vi "Position_Two_ScoringB.vi"(11 "data string":string) -> (3 "String":string)   [LabVIEW 2012, in "Serenity_mk2.lvrbt"]
uses:
  Serenity_mk2.lvrbt
  auto_drive_TYP.ctl
  State_Typ.ctl
  <vilib>/NXT/Dual Mode Library/Sound/Tone.vi
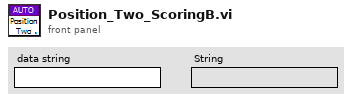
[diagram p1: front panel]
types:
  T1 = typedef "auto_drive_TYP.ctl" = cluster{"Left X":i8, "Left Y":i8, "Right Y":i8, "Power (100)":i8, "Wait (ms)":u32, "Enc/Deg Target":i32, "Move Type":enum16{"Relative Degrees", "Wait", "Encoder"}}
  T2 = typedef "State_Typ.ctl" = enum16{"Stop", "Check for Position 3", "Check for Position 2", "Move", "Reset Enc", "Read Enc", "Lift", "Dump Close"}
  T3 = typedef "LVHSConnector.ctl" = refnum<class "BrickReference.lvclass">
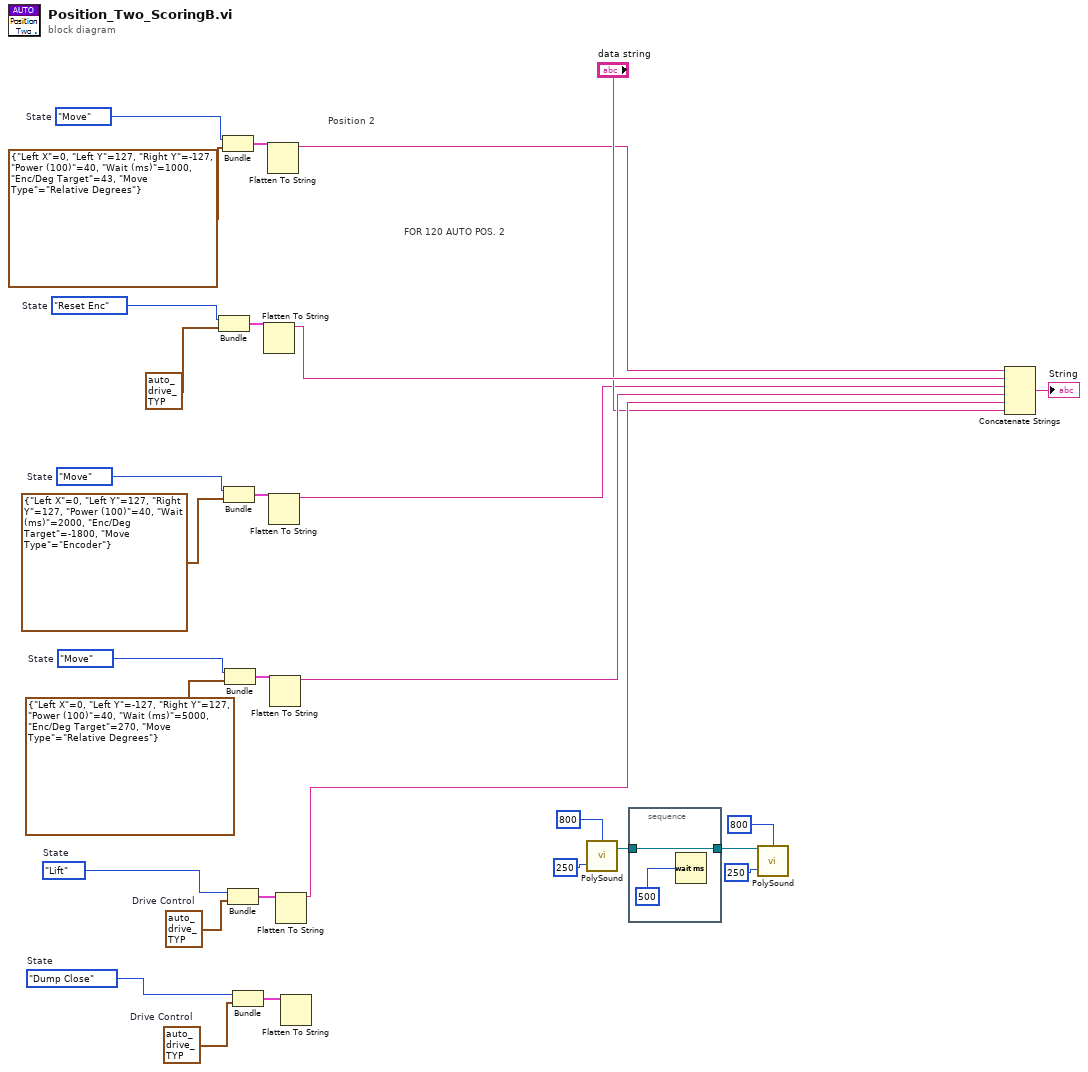
[diagram p0: block diagram]
diagram:
  w12 = T1 {"Left X"=0, "Left Y"=0, "Right Y"=0, "Power (100)"=100, "Wait (ms)"=3000, "Enc/Deg Target"=8450, "Move Type"=enum."Encoder"}  # Drive Control
  w13 = T1 {"Left X"=0, "Left Y"=0, "Right Y"=0, "Power (100)"=40, "Wait (ms)"=0, "Enc/Deg Target"=-6500, "Move Type"=enum."Encoder"}  # Drive Control
  w26 = State_Typ."Reset Enc"  # State
  w14 = State_Typ."Dump Close"  # State
  w10 = State_Typ."Lift"  # State
  w9 = State_Typ."Move"  # State
  w6 = State_Typ."Move"  # State
  w3 = State_Typ."Move"  # State
  # "FOR 120 AUTO POS. 2"
  # "Position 2"
  n1 = Bundle("State"=w26, "Drive Control"=T1 {"Left X"=0, "Left Y"=127, "Right Y"=127, "Power (100)"=40, "Wait (ms)"=2000, "Enc/Deg Target"=1800, "Move Type"=enum."Encoder"}) -> (w25:cluster{"State":T2, "Drive Control":T1})  [unwired: 1 in]
  n2 = Bundle("State"=w3, "Drive Control"=T1 {"Left X"=0, "Left Y"=127, "Right Y"=-127, "Power (100)"=40, "Wait (ms)"=1000, "Enc/Deg Target"=43, "Move Type"=enum."Relative Degrees"}) -> (w2:cluster{"State":T2, "Drive Control":T1})  [unwired: 1 in]
  n3 = Bundle("State"=w6, "Drive Control"=T1 {"Left X"=0, "Left Y"=127, "Right Y"=127, "Power (100)"=40, "Wait (ms)"=2000, "Enc/Deg Target"=-1800, "Move Type"=enum."Encoder"}) -> (w5:cluster{"State":T2, "Drive Control":T1})  [unwired: 1 in]
  n4 = Bundle("State"=w9, "Drive Control"=T1 {"Left X"=0, "Left Y"=-127, "Right Y"=127, "Power (100)"=40, "Wait (ms)"=5000, "Enc/Deg Target"=270, "Move Type"=enum."Relative Degrees"}) -> (w8:cluster{"State":T2, "Drive Control":T1})  [unwired: 1 in]
  n5 = Bundle("State"=w10, "Drive Control"=w12) -> (w11:cluster{"State":T2, "Drive Control":T1})  [unwired: 1 in]
  n6 = Bundle("State"=w14, "Drive Control"=w13) -> (w18:cluster{"State":T2, "Drive Control":T1})  [unwired: 1 in]
  n7 = Flatten To String(anything=w25) -> (data string=w27:string)  [unwired: 3 in, 2 out]
  n8 = Flatten To String(anything=w2) -> (data string=w16:string)  [unwired: 3 in, 2 out]
  n9 = Flatten To String(anything=w5) -> (data string=w17:string)  [unwired: 3 in, 2 out]
  n10 = Flatten To String(anything=w8) -> (data string=w28:string)  [unwired: 3 in, 2 out]
  n11 = Flatten To String(anything=w11) -> (data string=w29:string)  [unwired: 3 in, 2 out]
  n12 = Flatten To String(anything=w18) -> ()  [unwired: 3 in, 3 out]
  n13 = call-poly <vilib>:"PolySound.vi"("Duration (500 ms)"=u16 250, "Tone (440 Hz)"=u16 800) -> ("NXT/EV3"=w31:T3)  [unwired: 2 in]
  n14 = stacked-sequence {
    tunnel: [w32] -> w30
    tunnel: w31 -> [w32]
    frame #0 {
      n15 = Wait (ms)(milliseconds to wait=u32 500 ("Time (1 sec)")) -> ()  [unwired: 1 out]
    }
  }
  n16 = call-poly <vilib>:"PolySound.vi"("Duration (500 ms)"=u16 250, "NXT/EV3"=w30, "Tone (440 Hz)"=u16 800) -> ()  [unwired: 1 in, 1 out]
  n17 = Concatenate Strings(w16, w27, w17, w28, w29, "data string") -> (→"String":string)
